vi "prepare client.vi"(8 "error in":errorcluster, 10 "connection string":string, 11 "connection client in":refnum<class "connection client.lvclass">) -> (0 "error out":errorcluster, 3 "connection client out":refnum<class "connection client.lvclass">)   [LabVIEW 2015, in "connection client.lvclass"]
uses:
  connection client.lvclass
  connection client.lvclass/connection client.ctl
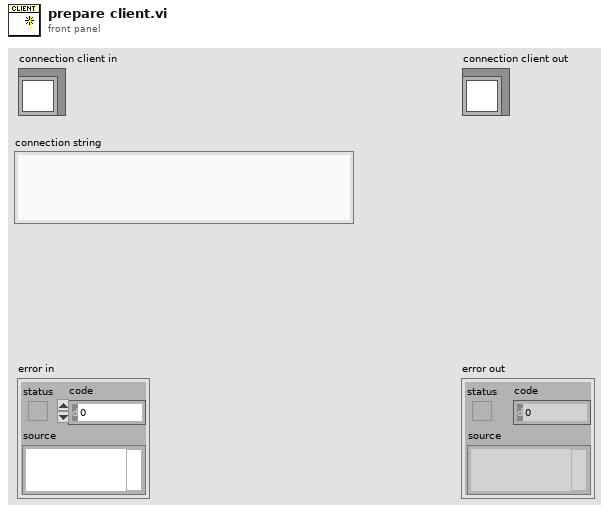
[diagram p1: front panel]
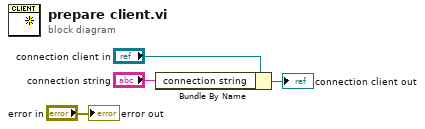
[diagram p0: block diagram]
diagram:
  n1 = Bundle By Name(cluster="connection client in", "connection string"="connection string") -> (→"connection client out":refnum<class "connection client.lvclass">)
  "error out" <- "error in"
